vi "licdf app decrypt.vi"(0 "handle":i32, 1 "out_cap":i32, 5 "packed":string, 7 "packed_len":i32, 9 "out":string, 11 "error in (no error)":errorcluster, 12 "out_len":i32) -> (4 "function return":i32, 10 "out out":string, 14 "out_len out":i32, 15 "error out":errorcluster)   [LabVIEW 2026, in "keynub_licdongle.lvlib"]
doc: "int32_t licdf_app_decrypt(int32_t handle, const uint8_t *packed, int32_t packed_len,\n uint8_t *out, int32_t out_cap, int32_t *out_len);"
uses:
  keynub_licdongle.lvlib
  natives/win-x64/keynub_licdongle_flat.dll
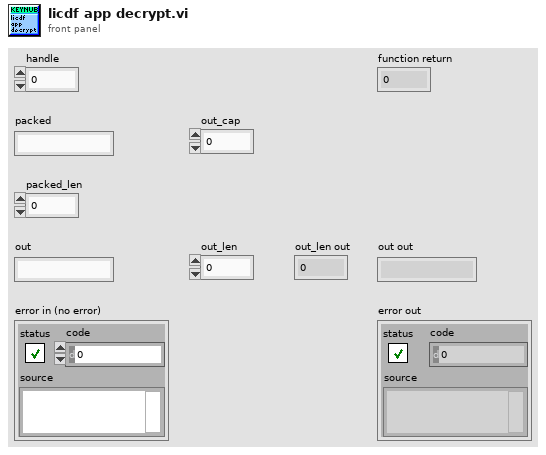
[diagram p1: front panel]
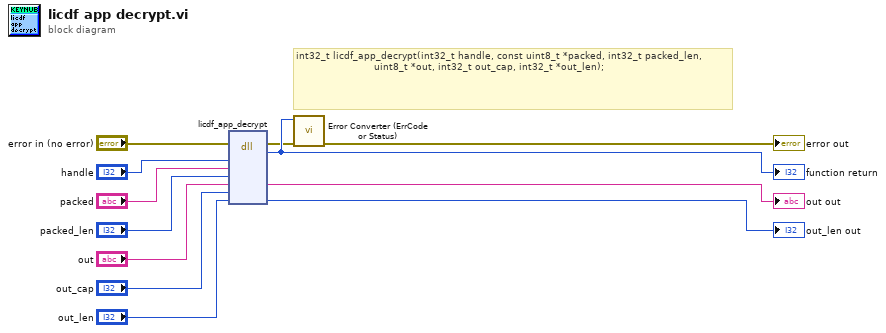
[diagram p0: block diagram]
diagram:
  # "int32_t licdf_app_decrypt(int32_t handle, const uint8_t *packed, int32_t packed_len,\n                          uint8_t *out, int32_t out_cap, int32_t *out_len);"
  n1 = dll-call lib="C:/Austausch/KeyNub/LicenseDongle-PublicSDK/natives/win-x64/keynub_licdongle_flat.*" fn="licdf_app_decrypt"(error in="error in (no error)", "handle"="handle", "packed"="packed", "packed_len"="packed_len", "out"="out", "out_cap"="out_cap", "out_len"="out_len") -> (error out=w2:errorcluster, w12:i32, "out"=→"out out":string, "out_len"=→"out_len out":i32)  [unwired: 6 in, 1 out]
  "function return" <- w12
  n2 = call "Error Converter (ErrCode or Status).vi"("error in (no error)"=w2, "error code"=w12) -> ("error out"=→"error out":errorcluster)  [unwired: 9 in]
